vi "Icon Editor Test.vi"() -> ()   [LabVIEW 2018]
uses:
  <vilib>/picture/picture.llb/imagedata.ctl
  class1/class1.lvclass
  <vilib>/LabVIEW Icon API/lv_icon/Classes/Icon/Icon.lvclass
  <vilib>/LabVIEW Icon API/API_Rectangle Dimension.ctl
  <vilib>/Utility/miscctls.llb/LVPoint32TypeDef.ctl
  <vilib>/LabVIEW Icon API/API_Text.ctl
  <vilib>/LabVIEW Icon API/API_Rectangle Colors.ctl
  <vilib>/LabVIEW Icon API/API_User Layer Data.ctl
  <vilib>/LabVIEW Icon API/lv_icon/Classes/Icon Framework/Icon Framework.lvclass
  <vilib>/LabVIEW Icon API/API_Test Settings.ctl
  <vilib>/LabVIEW Icon API/lv_icon/Controls/Alignment.ctl
  <vilib>/LabVIEW Icon API/API_Text Colors.ctl
  <vilib>/LabVIEW Icon API/LabVIEW Icon API.lvlib
panel:
  out "error out":errorcluster
  out "Color 256":T1
  out "2D Picture":picture
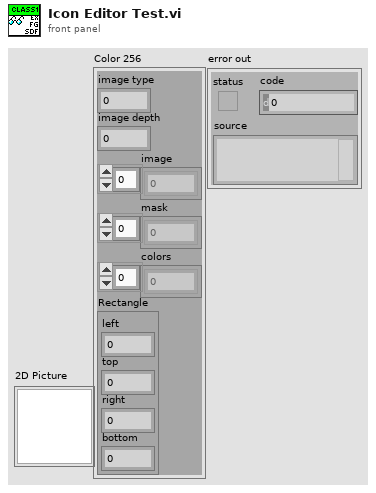
[diagram p1: front panel]
types:
  T1 = typedef "imagedata.ctl" = cluster{"image type":i32, "image depth":i32, "image":u8[], "mask":u8[], "colors":u32[], "Rectangle":cluster{"left":i16, "top":i16, "right":i16, "bottom":i16}}
  T2 = typedef "LabVIEW Icon API.lvlib/API_Test Settings.ctl" = cluster{"Font":string, "Alignment":T3, "Size":u8, "Center text":bool, "Capitalize text":bool, "Text color":T4}
  T3 = typedef "Alignment.ctl" = u16
  T4 = typedef "LabVIEW Icon API.lvlib/API_Text Colors.ctl" = cluster{"Line 1 color":u32, "Line 2 color":u32, "Line 3 color":u32, "Line 4 color":u32}
  T5 = typedef "LVPoint32TypeDef.ctl" = cluster{"Horizontal":i32, "Vertical":i32}
  T6 = typedef "LabVIEW Icon API.lvlib/API_User Layer Data.ctl" = cluster{"Layer name":string, "Origin":T5, "Icon image data":T1}
  T7 = cluster{"left":i16, "top":i16, "right":i16, "bottom":i16}
  T8 = typedef "LabVIEW Icon API.lvlib/API_Rectangle Colors.ctl" = cluster{"Border":u32, "Background":u32}
  T9 = typedef "LabVIEW Icon API.lvlib/API_Text.ctl" = cluster{"Line 1 text":string, "Line 2 text":string, "Line 3 text":string, "Line 4 text":string}
  T10 = typedef "LabVIEW Icon API.lvlib/API_Rectangle Dimension.ctl" = cluster{"Width":i16, "Height":i16}
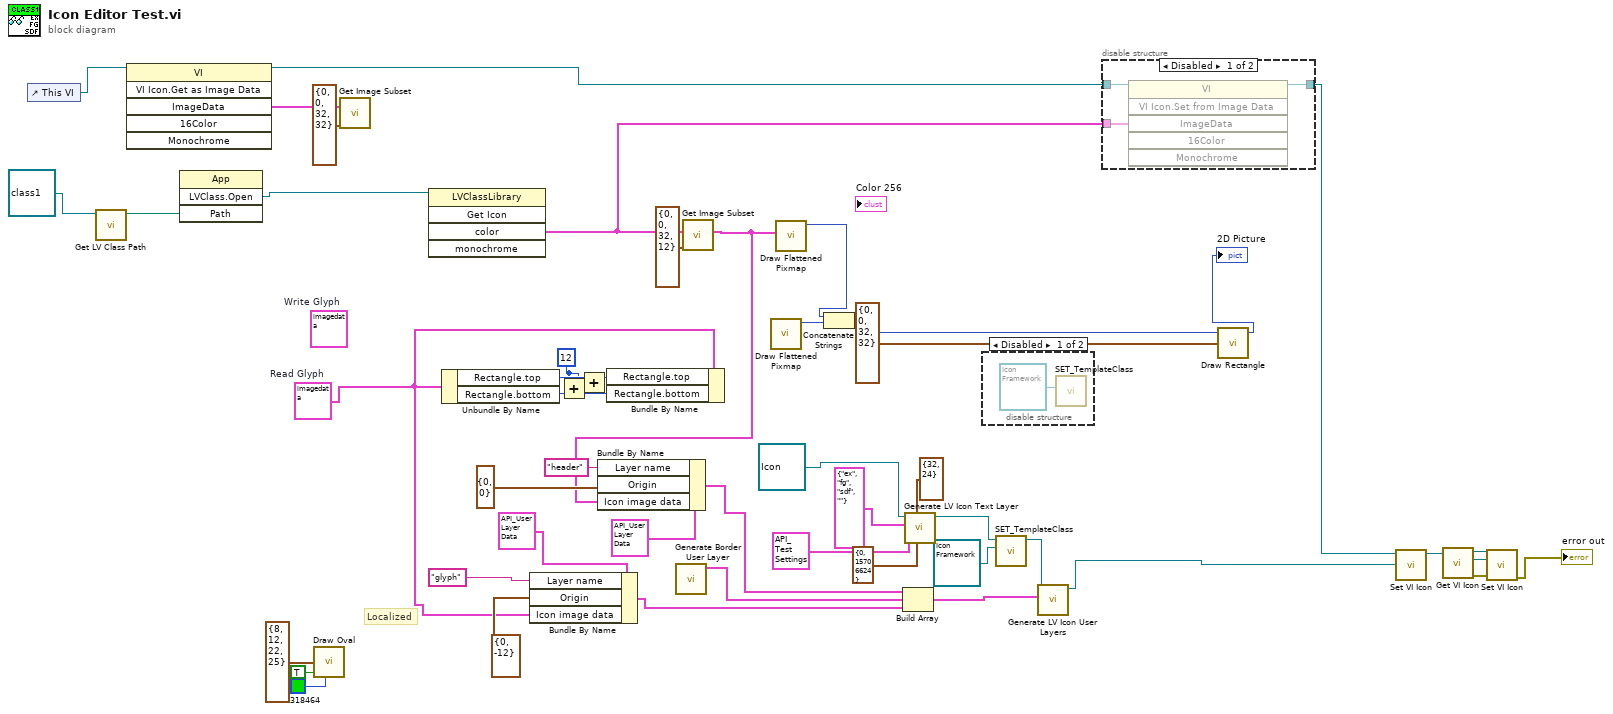
[diagram p0: block diagram]
diagram:
  w33 = i16 12 ("bottom")
  (unwired) T1 {"image type"=0, "image depth"=8, "image"=[0, 0, 0, 0, 0, 0, 0, 0, 0, 179, 0, 0, 0, 0, 0, 0, 0, 0, 0, 0, 0, 0, 179, 35, 107, 0, 0, 0, 0, 0, 0, 0, 0, 0, 0, 179, 107, 35, 35, 107, 0, 0, 0, 0, 0, 0, 0, 0, 179, 250, 250, 107, 35, 35, 179, 0, 0, 0, 0, 0, 0, 179, 5, 252, 250, 250, 107, 179, 0, 0, 0, 0, 0, 0, 179, 5, 1, 46, 252, 250, 179, 0, 0, 0, 0, 0, 0, 179, 5, 1, 46, 95, 95, 179, 0, 0, 0, 0, 0, 0, 179, 5, 1, 46, 95, 95, 179, 0, 0, 0, 0, 0, 0, 0, 179, 179, 46, 95, 95, 179, 0, 0, 0, 0, 0, 0, 0, 179, 0, 0, 179, 95, 179, 0, 0, 0, 0, 0, 0, 0, 0, 179, 0, 0, 179, 179, 0, 0, 0, 0, 0, 0, 0, 0, 255, 255, 179, 179, 0, 0, 0, 0, 0, 0, 0, 0, 0, 0, 255, 255, 0, 0, 0, 0, 0, 0, 0, 0, 0, 0, 0, 0], "mask"=[0, 64, 0, 224, 1, 240, 3, 248, 7, 240, 15, 224, 31, 192, 63, 128, 63, 0, 126, 0, 124, 0, 240, 0, 192, 0], "colors"=[16777215, 16777164, 16777113, 16777062, 16777011, 16776960, 16764159, 16764108, 16764057, 16764006, 16763955, 16763904, 16751103, 16751052, 16751001, 16750950, 16750899, 16750848, 16738047, 16737996, 16737945, 16737894, 16737843, 16737792, 16724991, 16724940, 16724889, 16724838, 16724787, 16724736, 16711935, 16711884, 16711833, 16711782, 16711731, 16711680, 13434879, 13434828, 13434777, 13434726, 13434675, 13434624, 13421823, 13421772, 13421721, 13421670, 13421619, 13421568, 13408767, 13408716, 13408665, 13408614, 13408563, 13408512, 13395711, 13395660, 13395609, 13395558, 13395507, 13395456, 13382655, 13382604, 13382553, 13382502, 13382451, 13382400, 13369599, 13369548, 13369497, 13369446, 13369395, 13369344, 10092543, 10092492, 10092441, 10092390, 10092339, 10092288, 10079487, 10079436, 10079385, 10079334, 10079283, 10079232, 10066431, 10066380, 10066329, 10066278, 10066227, 10066176, 10053375, 10053324, 10053273, 10053222, 10053171, 10053120, 10040319, 10040268, 10040217, 10040166, 10040115, 10040064, 10027263, 10027212, 10027161, 10027110, 10027059, 10027008, 6750207, 6750156, 6750105, 6750054, 6750003, 6749952, 6737151, 6737100, 6737049, 6736998, 6736947, 6736896, 6724095, 6724044, 6723993, 6723942, 6723891, 6723840, 6711039, 6710988, 6710937, 6710886, 6710835, 6710784, 6697983, 6697932, 6697881, 6697830, 6697779, 6697728, 6684927, 6684876, 6684825, 6684774, 6684723, 6684672, 3407871, 3407820, 3407769, 3407718, 3407667, 3407616, 3394815, 3394764, 3394713, 3394662, 3394611, 3394560, 3381759, 3381708, 3381657, 3381606, 3381555, 3381504, 3368703, 3368652, 3368601, 3368550, 3368499, 3368448, 3355647, 3355596, 3355545, 3355494, 3355443, 3355392, 3342591, 3342540, 3342489, 3342438, 3342387, 3342336, 65535, 65484, 65433, 65382, 65331, 65280, 52479, 52428, 52377, 52326, 52275, 52224, 39423, 39372, 39321, 39270, 39219, 39168, 26367, 26316, 26265, 26214, 26163, 26112, 13311, 13260, 13209, 13158, 13107, 13056, 255, 204, 153, 102, 51, 15597568, 14483456, 12255232, 11141120, 8912896, 7798784, 5570560, 4456448, 2228224, 1114112, 60928, 56576, 47872, 43520, 34816, 30464, 21760, 17408, 8704, 4352, 238, 221, 187, 170, 136, 119, 85, 68, 34, 17, 15658734, 14540253, 12303291, 11184810, 8947848, 7829367, 5592405, 4473924, 2236962, 1118481, 0], "Rectangle"={"left"=0, "top"=0, "right"=13, "bottom"=13}}  # Write Glyph
  w14 = T1 {"image type"=0, "image depth"=8, "image"=[0, 0, 0, 0, 0, 255, 255, 0, 0, 0, 0, 0, 0, 255, 255, 0, 0, 0, 0, 0, 255, 0, 0, 255, 0, 0, 0, 0, 255, 0, 0, 255, 0, 0, 0, 255, 0, 0, 0, 255, 0, 0, 0, 255, 0, 0, 0, 255, 0, 0, 255, 255, 0, 0, 0, 0, 0, 0, 255, 255, 0, 0, 0, 0, 0, 255, 0, 0, 255, 0, 255, 255, 0, 255, 0, 180, 255, 0, 0, 0, 255, 0, 0, 180, 180, 255, 0, 0, 255, 0, 0, 0, 180, 255, 0, 0, 255, 180, 0, 180, 187, 255, 0, 0, 255, 180, 0, 180, 187, 255, 0, 0, 0, 255, 180, 180, 255, 0, 0, 0, 0, 255, 180, 187, 255, 0, 0, 0, 0, 0, 255, 255, 0, 0, 0, 0, 0, 0, 255, 255, 0, 0, 0, 0, 0, 0, 0, 0, 0, 0, 0, 0, 0, 0, 0, 0, 0, 0, 0, 0], "mask"=[6, 6, 9, 9, 17, 17, 48, 48, 123, 120, 252, 252, 252, 252, 120, 120, 48, 48, 0, 0], "colors"=[16777215, 16777164, 16777113, 16777062, 16777011, 16776960, 16764159, 16764108, 16764057, 16764006, 16763955, 16763904, 16751103, 16751052, 16751001, 16750950, 16750899, 16750848, 16738047, 16737996, 16737945, 16737894, 16737843, 16737792, 16724991, 16724940, 16724889, 16724838, 16724787, 16724736, 16711935, 16711884, 16711833, 16711782, 16711731, 16711680, 13434879, 13434828, 13434777, 13434726, 13434675, 13434624, 13421823, 13421772, 13421721, 13421670, 13421619, 13421568, 13408767, 13408716, 13408665, 13408614, 13408563, 13408512, 13395711, 13395660, 13395609, 13395558, 13395507, 13395456, 13382655, 13382604, 13382553, 13382502, 13382451, 13382400, 13369599, 13369548, 13369497, 13369446, 13369395, 13369344, 10092543, 10092492, 10092441, 10092390, 10092339, 10092288, 10079487, 10079436, 10079385, 10079334, 10079283, 10079232, 10066431, 10066380, 10066329, 10066278, 10066227, 10066176, 10053375, 10053324, 10053273, 10053222, 10053171, 10053120, 10040319, 10040268, 10040217, 10040166, 10040115, 10040064, 10027263, 10027212, 10027161, 10027110, 10027059, 10027008, 6750207, 6750156, 6750105, 6750054, 6750003, 6749952, 6737151, 6737100, 6737049, 6736998, 6736947, 6736896, 6724095, 6724044, 6723993, 6723942, 6723891, 6723840, 6711039, 6710988, 6710937, 6710886, 6710835, 6710784, 6697983, 6697932, 6697881, 6697830, 6697779, 6697728, 6684927, 6684876, 6684825, 6684774, 6684723, 6684672, 3407871, 3407820, 3407769, 3407718, 3407667, 3407616, 3394815, 3394764, 3394713, 3394662, 3394611, 3394560, 3381759, 3381708, 3381657, 3381606, 3381555, 3381504, 3368703, 3368652, 3368601, 3368550, 3368499, 3368448, 3355647, 3355596, 3355545, 3355494, 3355443, 3355392, 3342591, 3342540, 3342489, 3342438, 3342387, 3342336, 65535, 65484, 65433, 65382, 65331, 65280, 52479, 52428, 52377, 52326, 52275, 52224, 39423, 39372, 39321, 39270, 39219, 39168, 26367, 26316, 26265, 26214, 26163, 26112, 13311, 13260, 13209, 13158, 13107, 13056, 255, 204, 153, 102, 51, 15597568, 14483456, 12255232, 11141120, 8912896, 7798784, 5570560, 4456448, 2228224, 1114112, 60928, 56576, 47872, 43520, 34816, 30464, 21760, 17408, 8704, 4352, 238, 221, 187, 170, 136, 119, 85, 68, 34, 17, 15658734, 14540253, 12303291, 11184810, 8947848, 7829367, 5592405, 4473924, 2236962, 1118481, 0], "Rectangle"={"left"=0, "top"=0, "right"=16, "bottom"=10}}  # Read Glyph
  # "Localized"
  n1 = control-ref of="This VI"() -> (w46:refnum<vi>)
  n2 = call <vilib>:"Get LV Class Path.vi"("object"=refnum<class "class1.lvclass"> refnum ("class1")) -> ("class path"=w48:path)  [unwired: 9 in, 1 out]
  n3 = invoke class="VI" method="VI Icon.Get as Image Data"(reference=w46) -> (reference out=w12:refnum<vi>, "ImageData"=w45:T1)  [unwired: 5 in, 4 out]
  n4 = invoke class="App" method="LVClass.Open"("Path"=w48) -> ("LVClass.Open"=w47:refnum<vi>)  [unwired: 3 in, 3 out]
  n5 = call <vilib>:"Draw Oval.vi"("rect"=T7 {"left"=8, "top"=12, "right"=22, "bottom"=25}, "fill?(F)"=TRUE, "color(black)"=u32 318464) -> ()  [unwired: 6 in, 1 out]
  n6 = call <vilib>:"Get Image Subset.vi"("subset rect"=T7 {"left"=0, "top"=0, "right"=32, "bottom"=32}, "image data"=w45) -> ()  [unwired: 4 in, 2 out]
  n7 = invoke class="LVClassLibrary" method="Get Icon"(reference=w47) -> ("color"=w16:T1)  [unwired: 4 in, 4 out]
  n8 = Unbundle By Name(w14) -> ("Rectangle.top"=w37:i16, "Rectangle.bottom"=w36:i16)
  n9 = Bundle By Name(cluster=T6 {"Layer name"="", "Origin"={"Horizontal"=0, "Vertical"=0}, "Icon image data"={"image type"=0, "image depth"=0, "image"=[], "mask"=[], "colors"=[], "Rectangle"={"left"=0, "top"=0, "right"=0, "bottom"=0}}} ("User layer"), "Layer name"="glyph", "Origin"=T5 {"Horizontal"=0, "Vertical"=-12}, "Icon image data"=w14) -> (w28:T6)
  n10 = Add(x=w33, y=w36) -> (x+y=w34:i16)
  n11 = Add(x=w37, y=w33) -> (x+y=w35:i16)
  n12 = Bundle By Name(cluster=w14, "Rectangle.top"=w35, "Rectangle.bottom"=w34) -> ()  [unwired: 1 out]
  n13 = call <vilib>:"Generate Border User Layer.vi"() -> ("User Layer data"=w24:T6)  [unwired: 11 in]
  n14 = call <vilib>:"Get Image Subset.vi"("subset rect"=T7 {"left"=0, "top"=0, "right"=32, "bottom"=12}, "image data"=w16) -> ("image subset"=w17:T1)  [unwired: 4 in, 1 out]
  n15 = Bundle By Name(cluster=T6 {"Layer name"="", "Origin"={"Horizontal"=0, "Vertical"=0}, "Icon image data"={"image type"=0, "image depth"=0, "image"=[], "mask"=[], "colors"=[], "Rectangle"={"left"=0, "top"=0, "right"=0, "bottom"=0}}} ("User layer"), "Layer name"="header", "Origin"=T5 {"Horizontal"=0, "Vertical"=0}, "Icon image data"=w17) -> (w15:T6)
  n16 = call <vilib>:"Draw Flattened Pixmap.vi"() -> ("new picture"=w42:picture)  [unwired: 9 in]
  n17 = call <vilib>:"Draw Flattened Pixmap.vi"("image data"=w17) -> ("new picture"=w41:picture)  [unwired: 8 in]
  n18 = Concatenate Strings(w41, w42) -> (w40:picture)
  n19 = Build Array(w15, w24, w28) -> (w27:T6[])
  n20 = call <vilib>:"Generate LV Icon Text Layer.vi"("Rectangle colors (black, white)"=T8 {"Border"=0, "Background"=15706624}, "Rectangle dimension (32,32)"=T10 {"Width"=32, "Height"=24}, "Text settings"=T2 {"Font"="Small Fonts", "Alignment"=2, "Size"=8, "Center text"=TRUE, "Capitalize text"=TRUE, "Text color"={"Line 1 color"=0, "Line 2 color"=0, "Line 3 color"=0, "Line 4 color"=0}}, "Text"=T9 {"Line 1 text"="ex", "Line 2 text"="fg", "Line 3 text"="sdf", "Line 4 text"=""}, "Icon in"=refnum<class "Icon.lvclass"> refnum ("Icon.lvclass in")) -> ("Icon out"=w8:refnum<class "Icon.lvclass">)  [unwired: 5 in, 1 out]
  n21 = disable-structure shown="Disabled" {
    frame Disabled {
      n22 = call-dynamic "SET_TemplateClass.vi"("Icon Framework.lvclass"=refnum<class "Icon Framework.lvclass"> refnum) -> ()  [unwired: 9 in, 2 out]
    }
    frame Enabled {
    }
  }
  n23 = call-dynamic "SET_TemplateClass.vi"("Icon Framework.lvclass"=refnum<class "Icon Framework.lvclass"> refnum, "Icon.lvclass in"=w8) -> ("Icon.lvclass out"=w7:refnum<class "Icon.lvclass">)  [unwired: 8 in, 1 out]
  n24 = call <vilib>:"Generate LV Icon User Layers.vi"("User layers"=w27, "Icon in"=w7) -> ("Icon out"=w10:refnum<class "Icon.lvclass">)  [unwired: 8 in, 1 out]
  n25 = disable-structure shown="Disabled" {
    disable-tunnel: w12 -> [w53 w54]
    disable-tunnel: w16 -> [w52 _]
    disable-tunnel: [w51 w54] -> w13
    frame Disabled {
      n26 = invoke class="VI" method="VI Icon.Set from Image Data"(reference=w53, "ImageData"=w52) -> (reference out=w51:refnum<vi>)  [unwired: 4 in, 5 out]
    }
    frame Enabled {
    }
  }
  n27 = call <vilib>:"Draw Rectangle.vi"("picture"=w40, "rect"=T7 {"left"=0, "top"=0, "right"=32, "bottom"=32}) -> ("new picture"=→"2D Picture":picture)  [unwired: 7 in]
  n28 = call <vilib>:"Set VI Icon.vi"("Icon"=w10, "VI Refnum in"=w13) -> ("VI Refnum out"=w6:refnum<vi>)  [unwired: 8 in, 1 out]
  n29 = call <vilib>:"Get VI Icon.vi"("VI Refnum in"=w6) -> ("error out"=w5:errorcluster, "Icon"=w4:refnum<class "Icon.lvclass">, "VI Refnum out"=w3:refnum<vi>)  [unwired: 8 in]
  n30 = call <vilib>:"Set VI Icon.vi"("error in (no error)"=w5, "Icon"=w4, "VI Refnum in"=w3) -> ("error out"=→"error out":errorcluster)  [unwired: 7 in, 1 out]
